vi "IdentifyBlob_Circle_Image.vi"(1 "color":u32(colorbox)=16773418, 2 "Centroid":cluster{"X":dbl, "Y":dbl}, 3 "Dimension":i32=10, 4 "picture":picture) -> (0 "picture":picture)   [LabVIEW 2024]
doc: "This VI is used with the BlobTracking.vi or the BiggestComplexBlob.vi. It will draw a shape centered on the blob's centroid. The shape depends upon the shape chosen by the poly selector and the dimension wired to the VI."
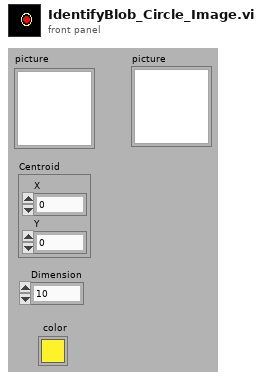
[diagram p1: front panel]
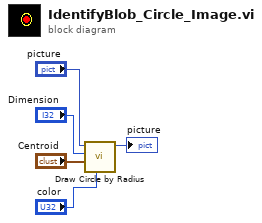
[diagram p0: block diagram]
diagram:
  n1 = call <vilib>:"Draw Circle by Radius.vi"("color(black)"="color", "pixel center"="Centroid", "radius"="Dimension", "picture"="picture") -> ("new picture"=→"picture":picture)  [unwired: 7 in]
